vi "Get DDGIOC Number Requested.vi"(11 "pulses":u32) -> (2 "function return":u32, 3 "pulses out":u32)   [LabVIEW 2018, in "Copy of Andor SDK.lvlib"]
doc: "EXPNETTYPE unsigned int WINAPI GetDDGIOCNumberRequested(at_u32 * pulses);"
uses:
  Copy of Andor SDK.lvlib
  <userlib>/Andor SDK/ATMCD32D.dll
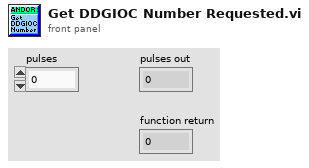
[diagram p1: front panel]
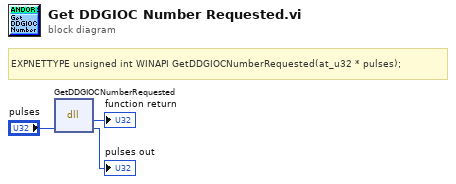
[diagram p0: block diagram]
diagram:
  # "EXPNETTYPE unsigned int WINAPI GetDDGIOCNumberRequested(at_u32 * pulses);"
  n1 = dll-call lib="C:/Program Files (x86)/National Instruments/LabVIEW 2018/user.lib/Andor SDK/ATMCD32D.*" fn="GetDDGIOCNumberRequested"("pulses"="pulses") -> (→"function return":u32, "pulses"=→"pulses out":u32)  [unwired: 3 in, 2 out]
